vi "PantherLAB_Log - Remove DQMH Event.vi"(10 "Event Info (Removed)":T1={"Event VI Path"=path "", "Argument Path"=path "", "Wait Argument Path"=path "", "Event Arg Owner"=-1, "Event Name"="", "Type"=enum."Request"}, 11 "Module Info":T3) -> (0 "error out":errorcluster)   [LabVIEW 2016]
doc: "_____\nCreated using DQMH Framework: Event Scripter 7.1.0.1450."
uses:
  <vilib>/Delacor/Delacor QMH/Libraries/_Scripting Support/Module Info--cluster.ctl
  <vilib>/Delacor/Delacor QMH/Libraries/_Scripting Support/Module Type--enum.ctl
  <vilib>/Delacor/Delacor QMH/Libraries/_Scripting Support/Event Info (Existing)--cluster.ctl
  Program Files (x86)/National Instruments/LabVIEW 2016/project/Delacor/DQMH/_DQMH Remove Event/Event Type (All Permutations)--enum.ctl
  PantherLAB Scripting Hooks/PantherLAB_Log.lvlib
  <vilib>/Delacor/Delacor QMH/Libraries/_Scripting Support/dqmh_lib_DQMH Scripting Support.lvlib
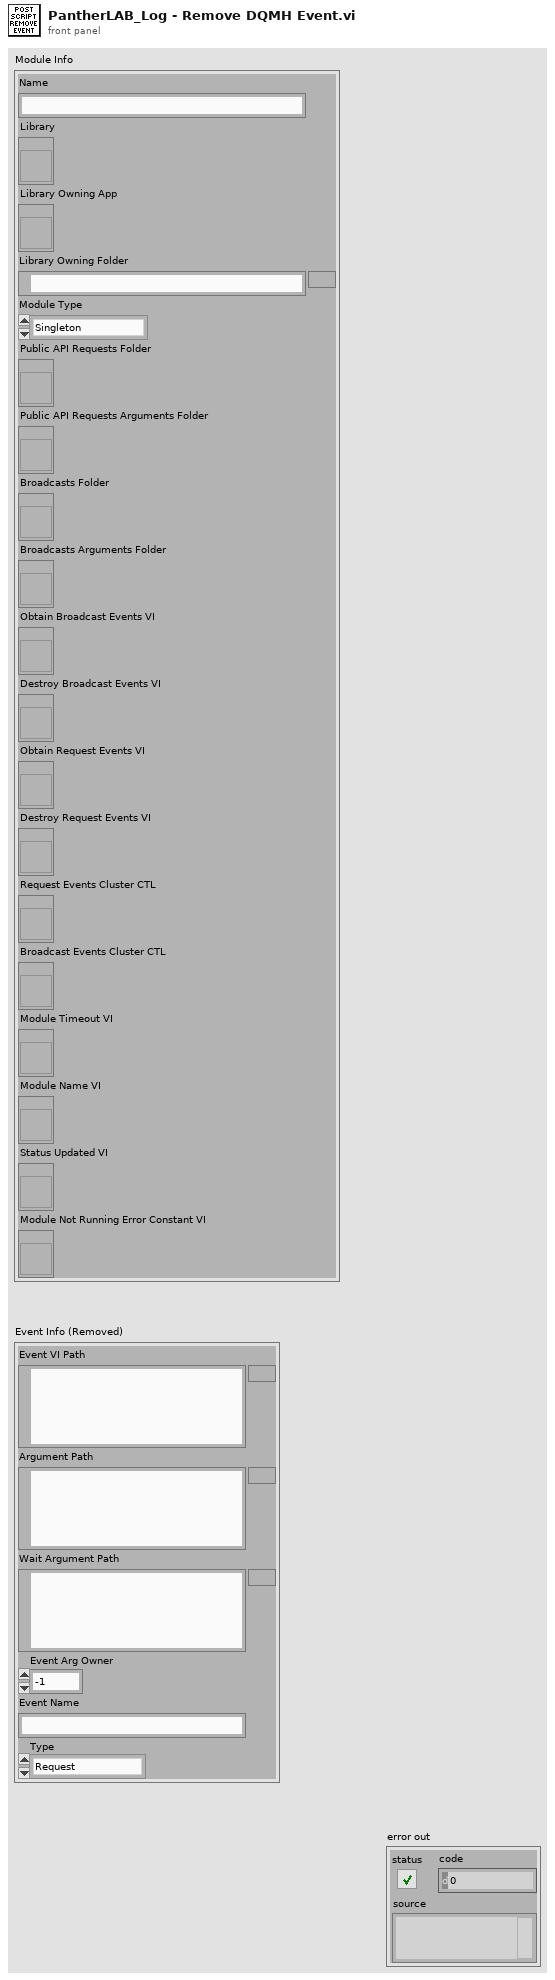
[diagram p1: front panel]
types:
  T1 = typedef "dqmh_lib_DQMH Scripting Support.lvlib/Event Info (Existing)--cluster.ctl" = cluster{"Event VI Path":path, "Argument Path":path, "Wait Argument Path":path, "Event Arg Owner":i32, "Event Name":string, "Type":T2}
  T2 = typedef "dqmh_lib_DQMH Scripting Support.lvlib/Event Type (All Permutations)--enum.ctl" = enum16{"Request", "Broadcast", "Both", "Request (no Wait)", "Request and Wait", "Request (Private)", "Request (Local Instance)"}
  T3 = typedef "dqmh_lib_DQMH Scripting Support.lvlib/Module Info--cluster.ctl" = cluster{"Name":string, "Library":refnum<vi>, "Library Owning App":refnum<vi>, "Library Owning Folder":path, "Module Type":T4, "Public API Requests Folder":refnum<vi>, "Public API Requests Arguments Folder":refnum<vi>, "Broadcasts Folder":refnum<vi>, "Broadcasts Arguments Folder":refnum<vi>, "Obtain Broadcast Events VI":refnum<vi>, "Destroy Broadcast Events VI":refnum<vi>, "Obtain Request Events VI":refnum<vi>, "Destroy Request Events VI":refnum<vi>, "Request Events Cluster CTL":refnum<vi>, "Broadcast Events Cluster CTL":refnum<vi>, "Module Timeout VI":refnum<vi>, "Module Name VI":refnum<vi>, "Status Updated VI":refnum<vi>, "Module Not Running Error Constant VI":refnum<vi>}
  T4 = typedef "dqmh_lib_DQMH Scripting Support.lvlib/Module Type--enum.ctl" = enum16{"Singleton", "Cloneable"}
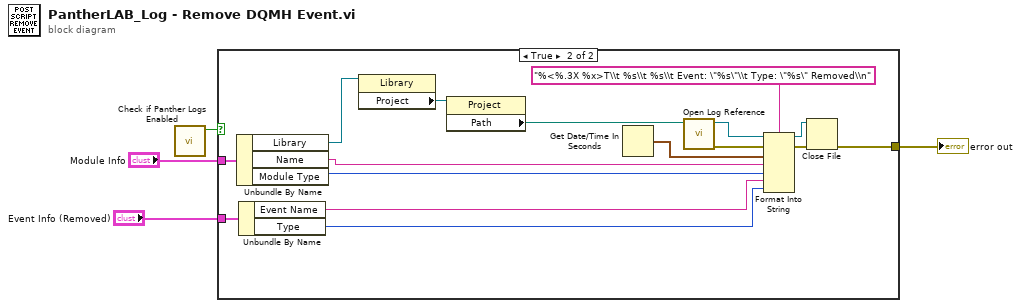
[diagram p0: block diagram]
diagram:
  n1 = call "Check if Panther Logs Enabled.vi"() -> ("PantherLogs Enabled?"=w3:bool)  [unwired: 11 in]
  n2 = case shown="True" w3 {
    tunnel: [_ w18] -> w4
    tunnel: "Module Info" -> [_ w17]
    tunnel: "Event Info (Removed)" -> [_ w8]
    frame False {
    }
    frame True {
      n3 = Unbundle By Name(w17) -> ("Library"=w16:refnum<vi>, "Name"=w12:string, "Module Type"=w11:T4)
      n4 = Unbundle By Name(w8) -> ("Event Name"=w7:string, "Type"=w6:T2)
      n5 = property class="Library"(reference=w16) -> ("Project"=w15:refnum<vi>)  [unwired: 1 in, 2 out]
      n6 = property class="Project"(reference=w15) -> ("Path"=w9:path)  [unwired: 1 in, 2 out]
      n7 = Get Date/Time In Seconds() -> (seconds since 1Jan1904=w10:timestamp)
      n8 = call "Open Log Reference.vi"("Project Path"=w9) -> ("error out"=w20:errorcluster, "File Reference"=w14:refnum<file>)  [unwired: 9 in]
      n9 = Format Into String(format string="%<%.3X %x>T\\t %s\\t %s\\t Event: \"%s\"\\t Type: \"%s\" Removed\\n", initial string=w14, error in=w20, w10, w12, w11, w7, w6) -> (resulting string=w13:refnum<file>, error out=w19:errorcluster)
      n10 = Close File(refnum=w13, error in=w19) -> (error out=w18:errorcluster)  [unwired: 1 out]
    }
  }
  "error out" <- w4
